vi "Get Outgoing Frames Info.vi"(0 "Device Reference in":T2 format="%.0x", 5 "error in (no error)":errorcluster) -> (14 "Enable Present?":bool[](array[boolean]), 15 "Enable Refs":T1[](array[typedef]) format="%.0x", 17 "Number of Signals Per Frame":i32[](array[numeric]), 18 "Started?":bool[](array[boolean]), 19 "error out":errorcluster)   [LabVIEW 2009, in "NI-XNET Custom Device.lvlib"]
doc: "This VI is used to get and parse more information about the outgoing frames. This is the information we need to create seperate sessions for each outgoing frame and to keep track of the enable/disable channel that turns the frame transmission on and off."
uses:
  NI-XNET Custom Device.lvlib
  <vilib>/NI VeriStand/Custom Device API/Custom Device Item Ref.ctl
  <vilib>/NI VeriStand/Custom Device API/Data Reference.ctl
  <vilib>/NI VeriStand/Custom Device API/Get Item Property (Boolean).vi
  <vilib>/NI VeriStand/Custom Device API/Data Access Type.ctl
  <vilib>/NI VeriStand/Custom Device API/Get Item Property (String).vi
  <vilib>/NI VeriStand/Custom Device API/Get Item Property (Variant).vi
  <vilib>/NI VeriStand/Custom Device API/Custom Device API.lvlib
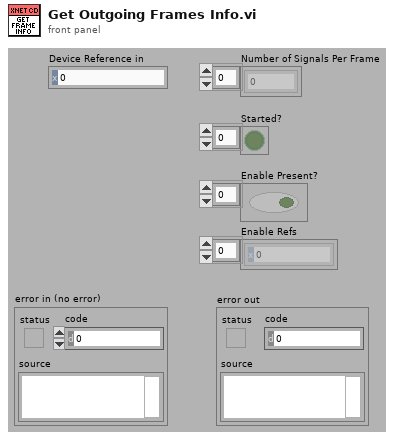
[diagram p1: front panel]
types:
  T1 = typedef "Custom Device API.lvlib/Data Reference.ctl" = i32
  T2 = typedef "Custom Device API.lvlib/Custom Device Item Ref.ctl" = u64
  T3 = typedef "Custom Device API.lvlib/Data Access Type.ctl" = enum16{"Read", "Write"}
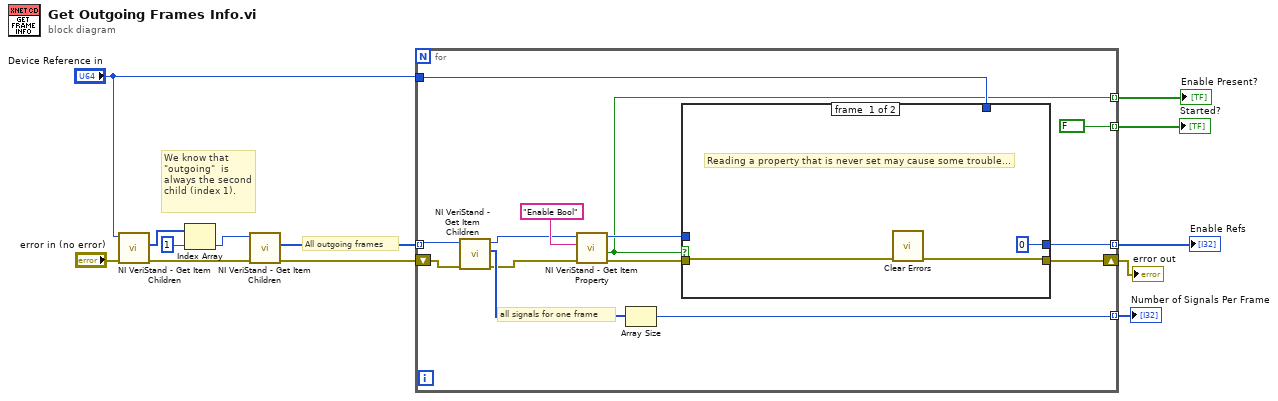
[diagram p0: block diagram]
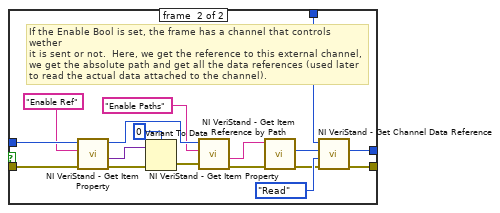
[diagram p2: hidden frame]
diagram:
  # "All outgoing frames"
  # "We know that \"outgoing\"  is always the second child (index 1)."
  n1 = call <vilib>:"NI VeriStand - Get Item Children.vi"("error in (no error)"="error in (no error)", "Item Ref in"="Device Reference in") -> ("error out"=w5:errorcluster, "Child Refs"=w9:T2[])  [unwired: 6 in, 2 out]
  n2 = Index Array(array=w9, index=1) -> (element=w8:T2)
  n3 = call <vilib>:"NI VeriStand - Get Item Children.vi"("error in (no error)"=w5, "Item Ref in"=w8) -> ("error out"=w4:errorcluster, "Child Refs"=w10:T2[])  [unwired: 6 in, 2 out]
  n4 = for {
    tunnel: w10 -> [w22] mode=indexing
    tunnel: [w16] -> w11 mode=indexing
    tunnel: [w24] -> w12 mode=indexing
    tunnel: "Device Reference in" -> [w25]
    tunnel: [w18] -> w2 mode=indexing
    shift-right: [w23] -> w3
    shift-left: w4 -> [w21]
    tunnel: [FALSE] -> w1 mode=indexing
    # "all signals for one frame"
    n5 = call <vilib>:"NI VeriStand - Get Item Children.vi"("error in (no error)"=w21, "Item Ref in"=w22) -> ("error out"=w17:errorcluster, "Child Refs"=w19:T2[], "Item Ref out"=w20:T2)  [unwired: 6 in, 1 out]
    n6 = call-poly <vilib>:"NI VeriStand - Get Item Property.vi"("error in (no error)"=w17, "Property Name"="Enable Bool", "Item Ref in"=w20) -> ("error out"=w15:errorcluster, "Value"=w16:bool, "Item Ref out"=w26:T2)  [unwired: 5 in, 1 out]
    n7 = Array Size(array=w19) -> (size(s)=w18:i32)
    n8 = case shown="True" w16 {
      tunnel: w26 -> [_ w47]
      tunnel: w25 -> [_ w39]
      tunnel: [T1 0 ("Channel Data Reference") w37] -> w24
      tunnel: [w29 w36] -> w23
      tunnel: w15 -> [w28 w33]
      frame #0 {
        # "Reading a property that is never set may cause some trouble..."
        n9 = call <vilib>:"Clear Errors.vi"("error in (no error)"=w28) -> ("error out"=w29:errorcluster)  [unwired: 6 in]
      }
      frame #1 {
        # "If the Enable Bool is set, the frame has a channel that controls wether \nit is sent or not.  Here, we get the reference to this external channel, we get the absolute path and get all the data references (used later to read the actual data attached to the channel)."
        n10 = call-poly <vilib>:"NI VeriStand - Get Item Property.vi"("error in (no error)"=w33, "Property Name"="Enable Ref", "Item Ref in"=w47) -> ("error out"=w32:errorcluster, "Value"=w45:variant, "Item Ref out"=w43:T2)  [unwired: 5 in, 1 out]
        n11 = Variant To Data(error in=w32, Variant=w45, type=T2 0 ("Channel Ref in")) -> (error out=w31:errorcluster)  [unwired: 1 out]
        n12 = call-poly <vilib>:"NI VeriStand - Get Item Property.vi"("error in (no error)"=w31, "Property Name"="Enable Paths", "Item Ref in"=w43) -> ("error out"=w34:errorcluster, "Value"=w41:string)  [unwired: 5 in, 2 out]
        n13 = call <vilib>:"NI VeriStand - Get Item Reference by Path.vi"("error in (no error)"=w34, "Item Path in"=w41) -> ("error out"=w35:errorcluster, "Item Ref"=w38:T2)  [unwired: 8 out]
        n14 = call <vilib>:"NI VeriStand - Get Channel Data Reference.vi"("error in (no error)"=w35, "Access"=Data_Access_Type."Read", "Channel Ref in"=w38, "Device Ref in"=w39) -> ("error out"=w36:errorcluster, "Channel Data Reference"=w37:T1)  [unwired: 6 out]
      }
    }
  }
  "Enable Refs" <- w12
  "Enable Present?" <- w11
  "error out" <- w3
  "Number of Signals Per Frame" <- w2
  "Started?" <- w1
